vi "produceTimingTicks.vi"(8 "error in (no error)":errorcluster, 10 "Channel":refnum<class "Channel.lvclass">, 11 "device in":refnum<class "device.lvclass">) -> (0 "error out":errorcluster, 3 "device out":refnum<class "device.lvclass">)   [LabVIEW 2009, in "Tools.lvlib" / "DatabaseHelpers.lvlib" / "device.lvclass"]
uses:
  device.lvclass
  Channel/Channel.lvclass
  device.lvclass/device.ctl
  Scripting/ScriptingEvent/ScriptEventList/ScriptEventList.lvclass
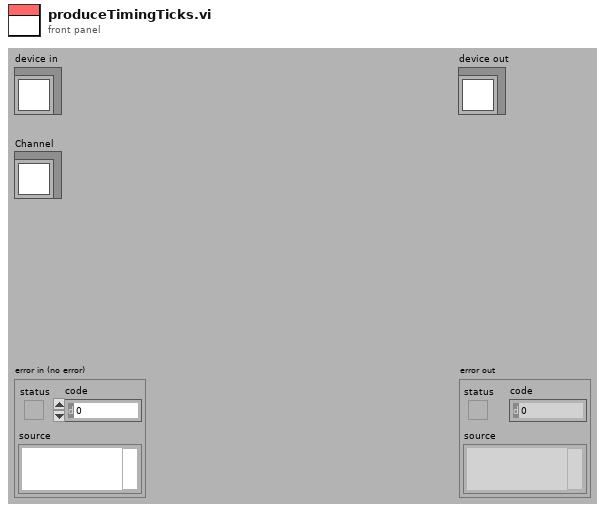
[diagram p1: front panel]
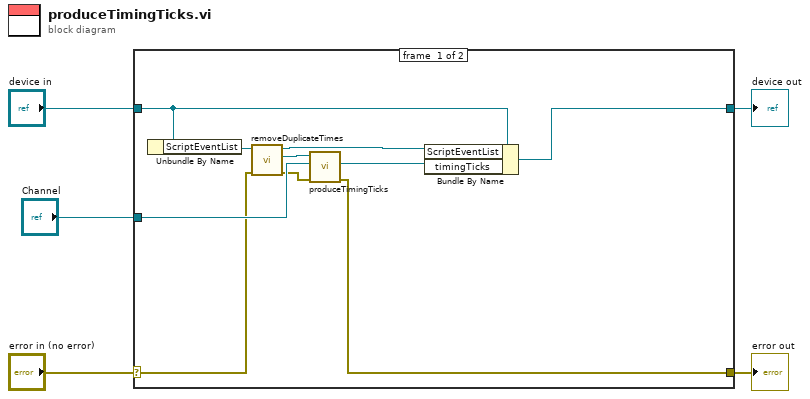
[diagram p0: block diagram]
diagram:
  n1 = case shown="No Error" "error in (no error)" {
    selector: "error in (no error)" -> [w7 w17]
    tunnel: [w14 w17] -> w4
    tunnel: [w11 w16] -> w2
    tunnel: "device in" -> [w12 w16]
    tunnel: "Channel" -> [w15 _]
    frame #0 {
      n2 = Unbundle By Name(w12) -> ("ScriptEventList"=w10:refnum<class "ScriptEventList.lvclass">)
      n3 = call "removeDuplicateTimes.vi"("error in (no error)"=w7, "ScriptEventList in"=w10) -> ("error out"=w6:errorcluster, "list"=w9:refnum<class "ScriptEventList.lvclass">, "ScriptEventList out"=w8:refnum<class "ScriptEventList.lvclass">)  [unwired: 7 in]
      n4 = call-dynamic "produceTimingTicks.vi"("error in (no error)"=w6, "Channel"=w15, "ScriptEventList in"=w9) -> ("error out"=w14:errorcluster, "timingTickList"=w13:refnum<class "ScriptEventList.lvclass">)  [unwired: 6 in, 1 out]
      n5 = Bundle By Name(cluster=w12, "ScriptEventList"=w8, "timingTicks"=w13) -> (w11:refnum<class "device.lvclass">)
    }
    frame #1 {
    }
  }
  "error out" <- w4
  "device out" <- w2
